vi "set.vi"(9 "values":string[](array[string])=["0", "hola", "3,25"], 10 "variables":string[](array[string])=["intin", "strinin", "time"], 11 "Experience ID":string="Test") -> (0 "error out":errorcluster={"status"=TRUE, "code"=1, "source"="Bad condversion\nWhile writing variable: intin\nOn expID:Test"})   [LabVIEW 2019]
panel:
  # "Set"
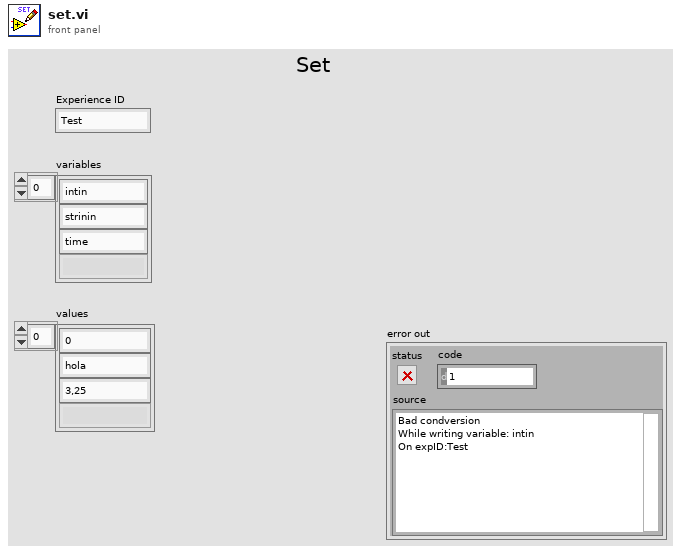
[diagram p1: front panel]
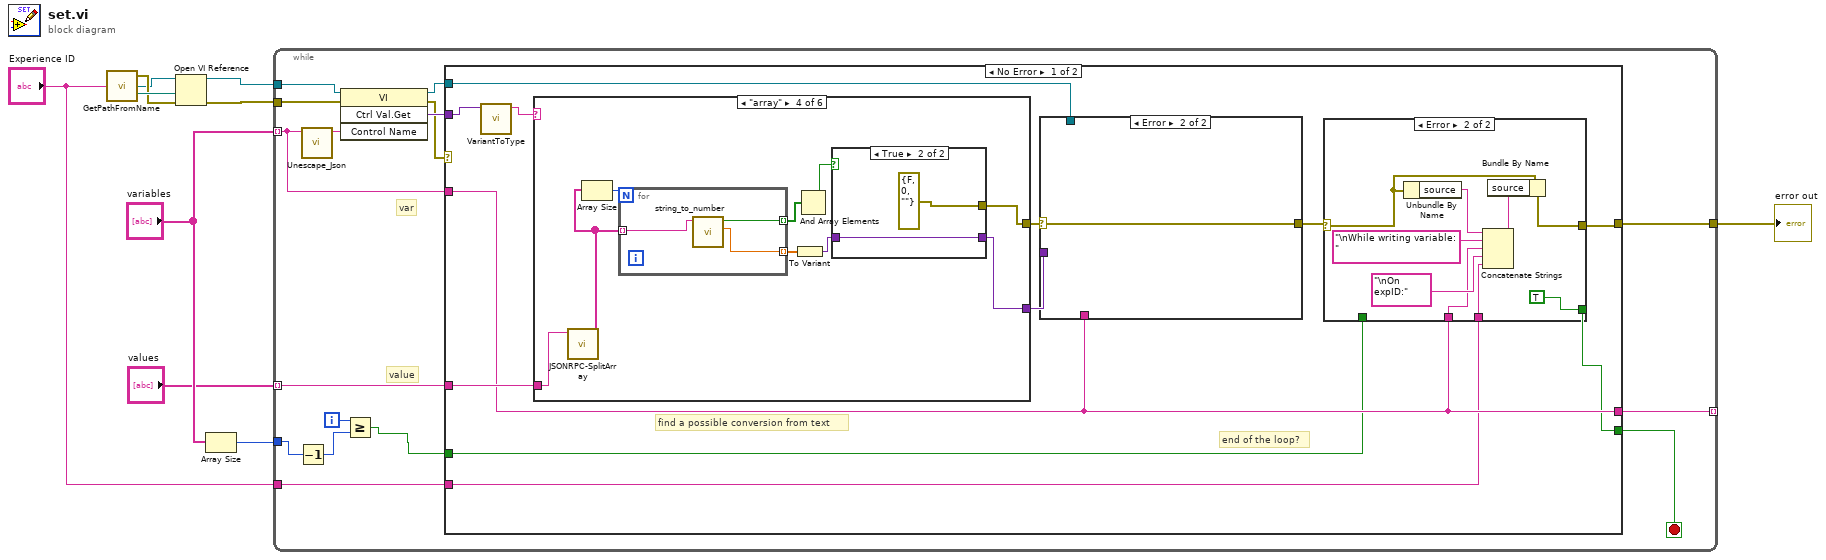
[diagram p0: block diagram]
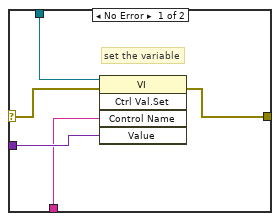
[diagram p3: hidden frame]
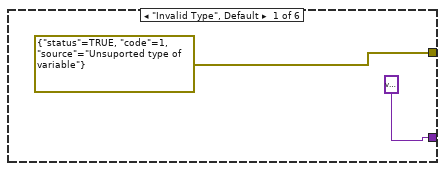
[diagram p4: hidden frame]
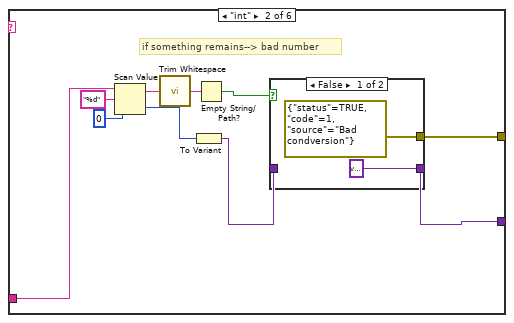
[diagram p5: hidden frame]
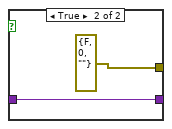
[diagram p6: hidden frame]
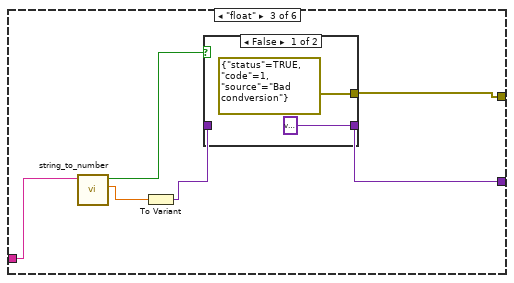
[diagram p7: hidden frame]
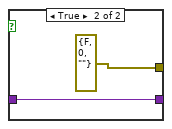
[diagram p8: hidden frame]
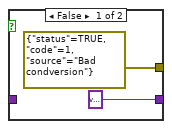
[diagram p9: hidden frame]
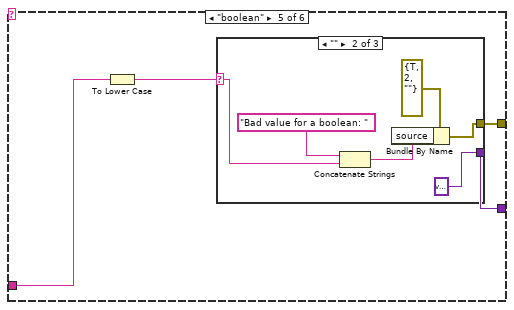
[diagram p10: hidden frame]
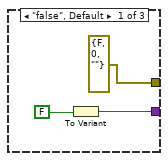
[diagram p11: hidden frame]
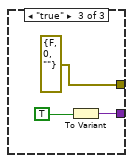
[diagram p12: hidden frame]
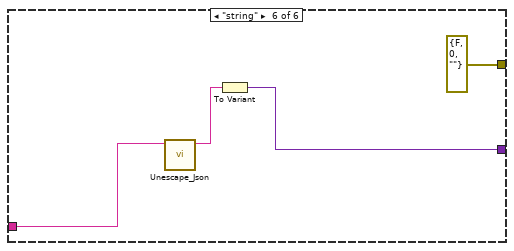
[diagram p13: hidden frame]
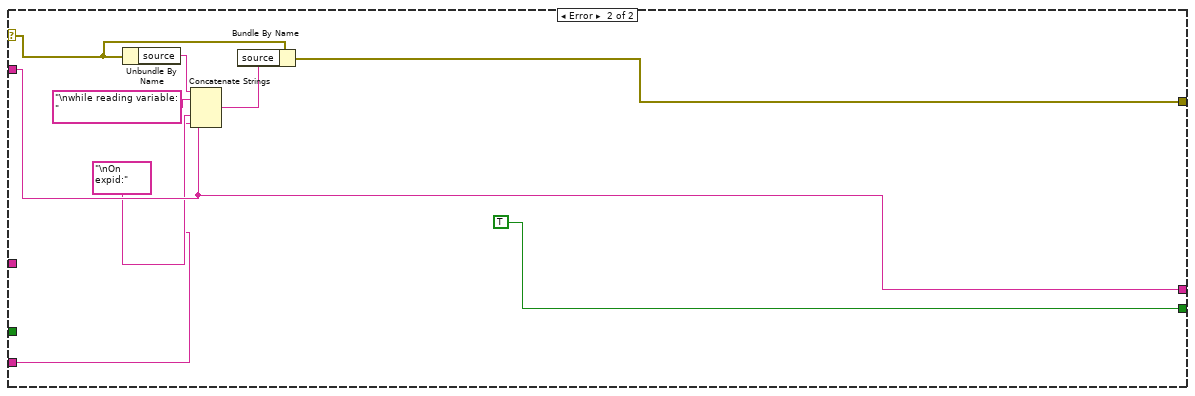
[diagram p14: hidden frame]
diagram:
  n1 = call "GetPathFromName.vi"("Experience ID"="Experience ID") -> ("VI_Path"=w10:path, "application reference"=w1:refnum<vi>, "Error out"=w9:errorcluster)  [unwired: 2 in]
  n2 = Open VI Reference(application reference (local)=w1, vi path=w10, error in (no error)=w9) -> (vi reference=w3:refnum<vi>, error out=w6:errorcluster)  [unwired: 3 out]
  n3 = Array Size(array="variables") -> (size(s)=w7:i32)
  n4 = while {
    tunnel: "variables" -> [w11] mode=indexing
    tunnel: w3 -> [w26]
    tunnel: w7 -> [w18]
    tunnel: w6 -> [w25]
    tunnel: [w21] -> w2
    tunnel: [w20] -> _ mode=indexing
    tunnel: "Experience ID" -> [w19]
    tunnel: "values" -> [w14] mode=indexing
    i -> [w16]
    stop <- w22 stop-if-true
    # "value"
    # "var"
    n5 = Decrement(x=w18) -> (x-1=w15:i32)
    n6 = call "Unescape_Json.vi"("Json_String"=w11) -> ("String"=w12:string)  [unwired: 9 in]
    n7 = invoke class="VI" method="Ctrl Val.Get"(reference=w26, error in=w25, "Control Name"=w12) -> (reference out=w13:refnum<vi>, error out=w23:errorcluster, "Get Control Value Variant"=w24:variant)  [unwired: 1 in, 1 out]
    n8 = Greater Or Equal?(x=w16, y=w15) -> (x >= y?=w17:bool)
    n9 = case shown="No Error" w23 {
      selector: w23 -> [_ w125]
      tunnel: w24 -> [w28 _]
      tunnel: w17 -> [w29 _]
      tunnel: [w30 TRUE] -> w22
      tunnel: w11 -> [w34 w120]
      tunnel: [w31 w121] -> w21
      tunnel: [w34 w120] -> w20
      tunnel: w19 -> [w33 w118]
      tunnel: w14 -> [w37 _]
      tunnel: w13 -> [w35 _]
      frame No Error {
        # "end of the loop?"
        # "find a possible conversion from text"
        n10 = call "VariantToType.vi"("Variant"=w28) -> ("type Name"=w27:string)  [unwired: 10 in]
        n11 = case shown="\"array\"" w27 {
          tunnel: [errorcluster {"status"=TRUE, "code"=1, "source"="Unsuported type of variable"} ("error out") w60 w76 w83 w100 errorcluster {"status"=FALSE, "code"=0, "source"=""} ("error IO")] -> w38
          tunnel: w37 -> [_ w67 w77 w89 w98 w114]
          tunnel: [variant ("Variant") w62 w75 w82 w101 w117] -> w36
          frame "Invalid Type", Default {
          }
          frame "int" {
            # "if something remains--> bad number"
            n12 = Scan Value(string=w67, format string="%d", default (0 dbl)=0) -> (output string=w58:string, value=w64:i32)
            n13 = call <vilib>:"Trim Whitespace.vi"("string"=w58) -> ("trimmed string"=w59:string)  [unwired: 1 in]
            n14 = To Variant(anything=w64) -> (Variant=w61:variant)
            n15 = Empty String/Path?(string/path=w59) -> (empty?=w63:bool)
            n16 = case shown="False" w63 {
              tunnel: [variant w71] -> w62
              tunnel: w61 -> [_ w71]
              tunnel: [errorcluster {"status"=TRUE, "code"=1, "source"="Bad condversion"} ("error IO") errorcluster {"status"=FALSE, "code"=0, "source"=""} ("error IO")] -> w60
              frame False {
              }
              frame True {
              }
            }
          }
          frame "float" {
            n17 = call "string_to_number.vi"("String"=w77) -> ("default (0 dbl)"=w72:dbl, "conversionOK"=w74:bool)  [unwired: 9 in]
            n18 = To Variant(anything=w72) -> (Variant=w73:variant)
            n19 = case shown="False" w74 {
              tunnel: [variant w81] -> w75
              tunnel: w73 -> [_ w81]
              tunnel: [errorcluster {"status"=TRUE, "code"=1, "source"="Bad condversion"} ("error IO") errorcluster {"status"=FALSE, "code"=0, "source"=""} ("error IO")] -> w76
              frame False {
              }
              frame True {
              }
            }
          }
          frame "array" {
            n20 = call "JSONRPC-SplitArray.vi"("input string"=w89) -> ("array"=w87:string[])  [unwired: 10 in]
            n21 = Array Size(array=w87) -> (size(s)=w88:i32)
            n22 = for {
              N: w88 -> [_]
              tunnel: w87 -> [w93] mode=indexing
              tunnel: [w92] -> w85 mode=indexing
              tunnel: [w91] -> w86 mode=indexing
              n23 = call "string_to_number.vi"("String"=w93) -> ("default (0 dbl)"=w91:dbl, "conversionOK"=w92:bool)  [unwired: 9 in]
            }
            n24 = To Variant(anything=w86) -> (Variant=w90:variant)
            n25 = And Array Elements(Boolean array=w85) -> (logical AND=w84:bool)
            n26 = case shown="True" w84 {
              tunnel: [variant w97] -> w82
              tunnel: w90 -> [_ w97]
              tunnel: [errorcluster {"status"=TRUE, "code"=1, "source"="Bad condversion"} ("error IO") errorcluster {"status"=FALSE, "code"=0, "source"=""} ("error IO")] -> w83
              frame False {
              }
              frame True {
              }
            }
          }
          frame "boolean" {
            n27 = To Lower Case(string=w98) -> (all lower case string=w99:string)
            n28 = case shown="\"\"" w99 {
              selector: w99 -> [_ w108 _]
              tunnel: [w103 variant ("Variant") w113] -> w101
              tunnel: [errorcluster {"status"=FALSE, "code"=0, "source"=""} ("error IO") w106 errorcluster {"status"=FALSE, "code"=0, "source"=""} ("error IO")] -> w100
              frame "false", Default {
                n29 = To Variant(anything=FALSE) -> (Variant=w103:variant)
              }
              frame "" {
                n30 = Concatenate Strings("Bad value for a boolean: " ("source"), w108) -> (w110:string)
                n31 = Bundle By Name(cluster=errorcluster {"status"=TRUE, "code"=2, "source"=""} ("error IO"), "source"=w110) -> (w106:errorcluster)
              }
              frame "true" {
                n32 = To Variant(anything=TRUE) -> (Variant=w113:variant)
              }
            }
          }
          frame "string" {
            n33 = call "Unescape_Json.vi"("Json_String"=w114) -> ("String"=w115:string)  [unwired: 9 in]
            n34 = To Variant(anything=w115) -> (Variant=w117:variant)
          }
        }
        n35 = case shown="Error" w38 {
          selector: w38 -> [w53 w55]
          tunnel: [w52 w55] -> w32
          tunnel: w34 -> [w50 _]
          tunnel: w36 -> [w51 _]
          tunnel: w35 -> [w54 _]
          frame No Error {
            # "set the variable"
            n36 = invoke class="VI" method="Ctrl Val.Set"(reference=w54, error in=w53, "Control Name"=w50, "Value"=w51) -> (error out=w52:errorcluster)  [unwired: 1 in, 4 out]
          }
          frame Error {
          }
        }
        n37 = case shown="Error" w32 {
          selector: w32 -> [w40 w47]
          tunnel: [w40 w48] -> w31
          tunnel: [w39 TRUE] -> w30
          tunnel: w34 -> [_ w42]
          tunnel: w33 -> [_ w41]
          tunnel: w29 -> [w39 _]
          frame No Error {
            # "ok"
          }
          frame Error {
            n38 = Unbundle By Name(w47) -> ("source"=w46:string)
            n39 = Concatenate Strings(w46, "\nWhile writing variable: " ("string"), w42, "\nOn expID:" ("string"), w41) -> (w44:string)
            n40 = Bundle By Name(cluster=w47, "source"=w44) -> (w48:errorcluster)
          }
        }
      }
      frame Error {
        n41 = Unbundle By Name(w125) -> ("source"=w124:string)
        n42 = Concatenate Strings(w124, "\nwhile reading variable: " ("string"), w120, "\nOn expid:", w118) -> (w122:string)
        n43 = Bundle By Name(cluster=w125, "source"=w122) -> (w121:errorcluster)
      }
    }
  }
  "error out" <- w2
